vi "Omniax_mDrive_Yonly_2017APXNoBK.vi"() -> ()   [LabVIEW 2015]
uses:
  <vilib>/Utility/file.llb/Read From Spreadsheet File (I64).vi
  <vilib>/Instr/_visa.llb/VISA Configure Serial Port (Instr).vi
  <userlib>/caLab/Private/Get_PV.vi
  Omniax_mDrive_GNDGlobal.vi
  <userlib>/caLab/Private/Put_DBL_PV.vi
  <vilib>/Utility/file.llb/Write To Spreadsheet File (I64).vi
  <vilib>/Utility/file.llb/Write To Spreadsheet File (string).vi
  <vilib>/Utility/file.llb/Read From Spreadsheet File (string).vi
panel:
  out "Z<350?":bool
  out "read buffer":string
  out "sample NC":bool
  in  "APX:MXYZR_STOP":bool
  in  "APX:MY_VLC_RQ":dbl min=0.0 max=0.1 step=0.01
  in  "APX:MY_RQ":dbl min=-3.0 max=2.0
  in  "Y Velocity SP step/sec":i32 min=1 max=12800
  in  "Y Step SP":i32=-20000 min=-2304000 max=2304000 step=500
  out "Y Step PV":i32 max=2000
  out "Boolean":bool
  out "PR P":string
  in  "V5 position 15360000":i32
  out "R Velocity MVdeg/sec":dbl format="%.3f"
  out "R Position MV deg":dbl
  out "Z Velocity MV mm/sec":dbl format="%.3f"
  out "Z Position MV mm":dbl
  out "Y Velocity MV mm/sec":dbl format="%.3f"
  out "Y Position MV mm":dbl
  out "X Velocity MV mm/sec":dbl format="%.3f"
  out "X Position MV mm":dbl
  out "Presets":i32[][](array[numeric])
  in  "stop":bool
  in  "Tab Control 3":enum32{"Status", "Reset"}(tab)
  out "APX:Y_LIM":bool
  out "APX:MY_MVG":bool
  out "APX:MY_RDY":bool
  in  "Reset Y Position mm":dbl
  out "Reset Y Motor Steps":i32
  in  "Reset":bool
  in  "Clear ZY":bool
  out "R Backlash steps/sec":i32
  out "R Backlash":i32
  out "R Holding Current %":i32
  out "R Run Current %":i32
  out "R velocity PV step/sec":i32
  out "Z Backlash steps/sec":i32
  out "Z Backlash":i32
  out "Z Holding Current %":i32
  out "Z Run Current %":i32
  out "Z  velocity PV step/sec":i32
  out "X velocity PV step/sec":i32
  out "X Backlash steps/sec":i32
  out "X Backlash":i32
  out "X Holding Current %":i32
  out "X Run Current %":i32
  out "Y Backlash steps/sec":i32
  out "Y Backlash":i32
  out "Y Holding Current %":i32
  out "Y Run Current %":i32
  out "APX:MY_PV":dbl
  out "Y offset mm":dbl
  out "Y mm/rev":dbl
  out "Y steps/rev":u32
  out "Y velocity PV step/sec":i32
  out "Y MINPOS":i32=-94296
  out "Y MAXPOS":i32=-34296
  out "Y COM PORT":refnum<visa-resource-name>="COM5"
  # "APX:MY"
  # "Goto position"
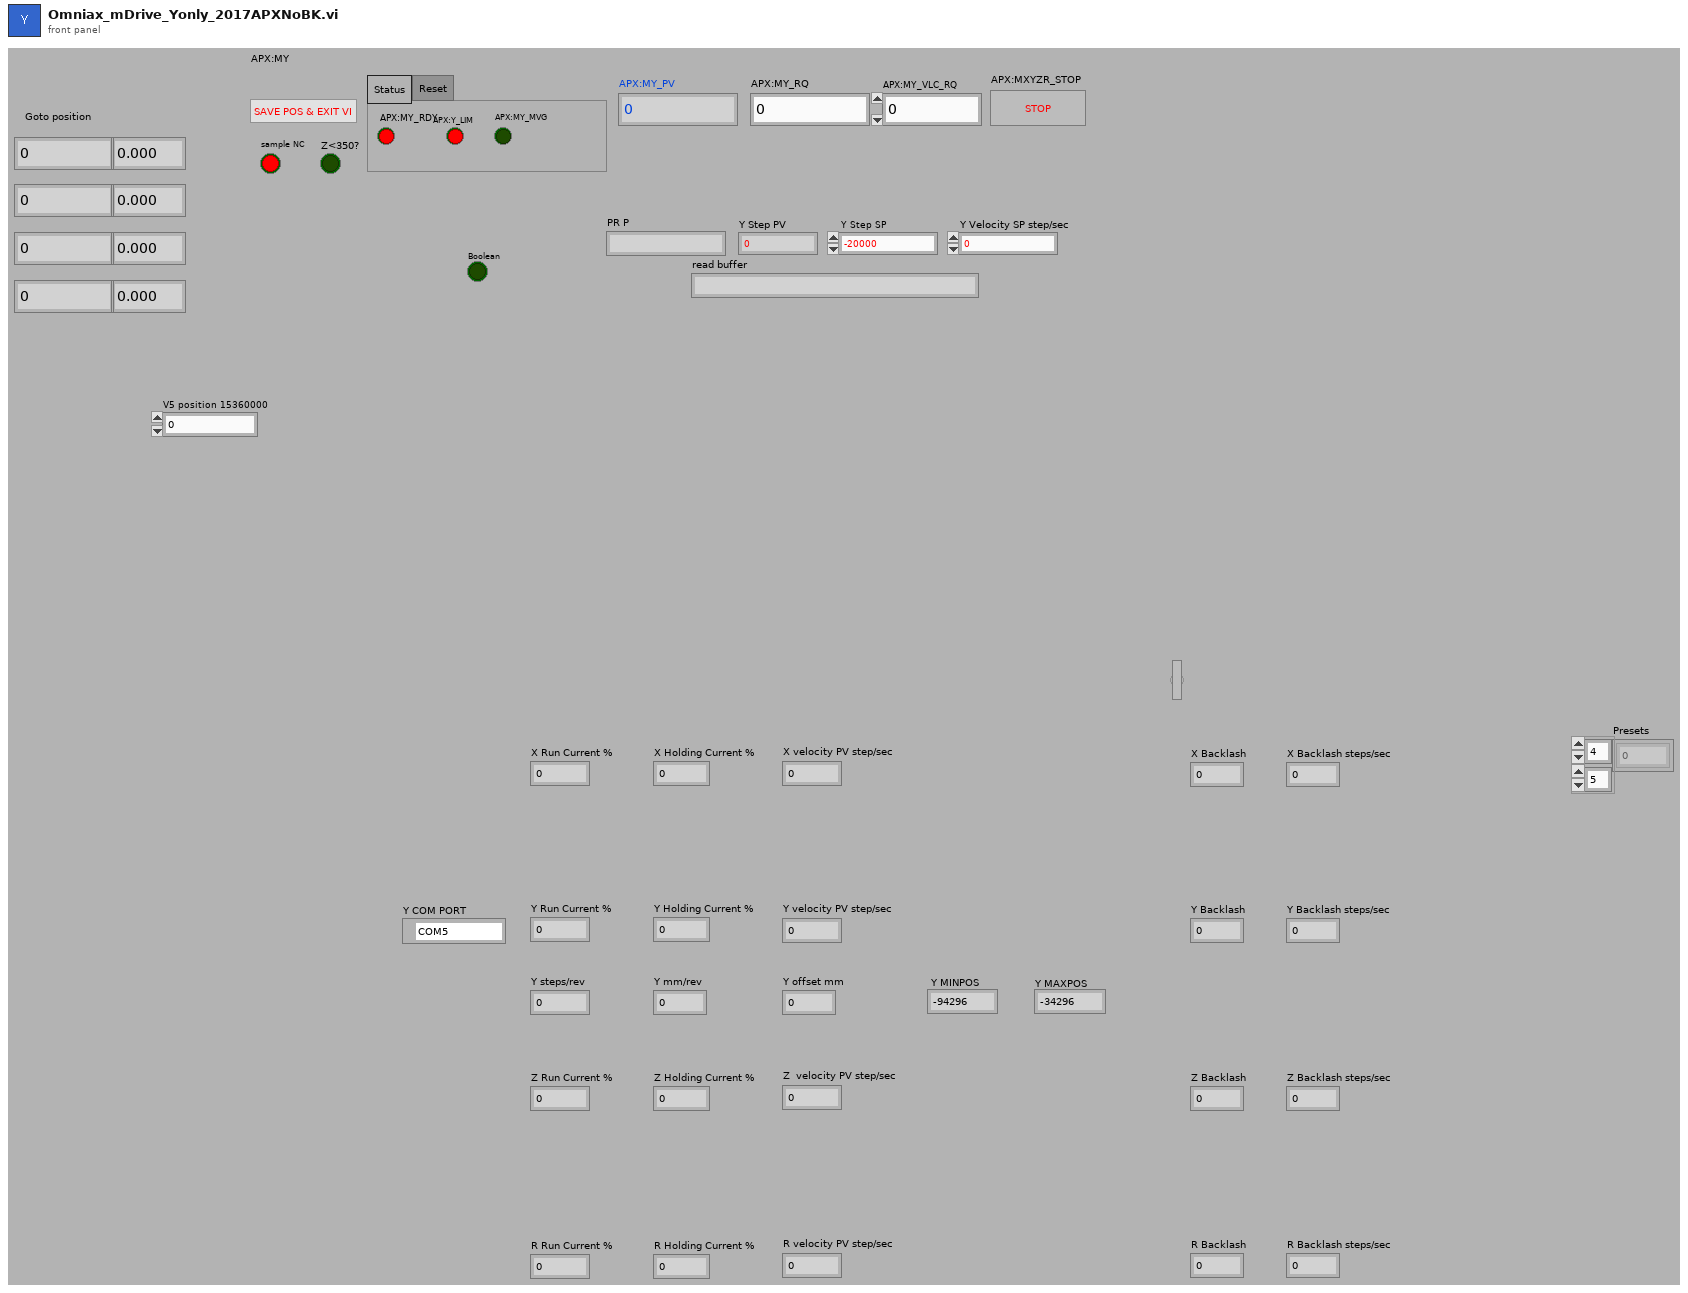
[diagram p1: front panel]
types:
  T1 = enum16{"Stop", "Reset", "Run Current", "Holding Current", "Accel Rate", "Decel Rate", "Move to Relative Position", "Move to Absolute Position", "Echo Mode", "Print Parameter", "Send String", "Microstep Resolution", "Set Current Position", "Max Velocity"}
  T2 = cluster{"first row[0]":i64, "first row[1]":i64, "first row[2]":i64, "first row[3]":i64, "first row[4]":i64, "first row[5]":i64, "first row[6]":i64, "first row[7]":i64, "first row[8]":i64}
  T3 = enum8{"Enabled", "Disabled", "Disabled and Grayed Out"}
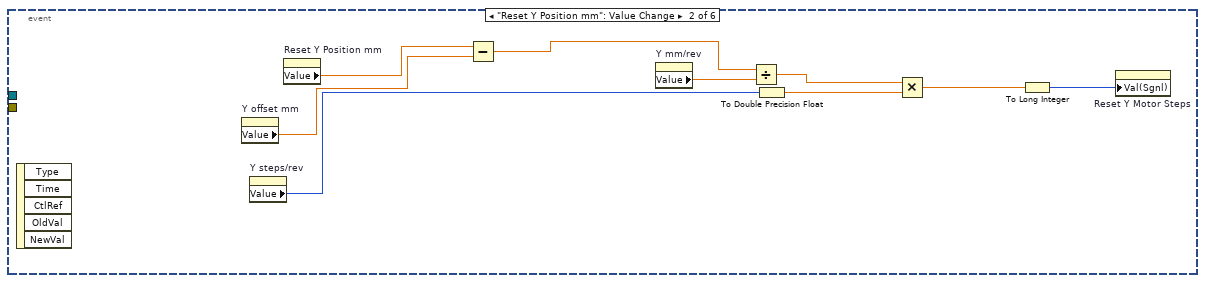
[diagram p13: hidden frame]
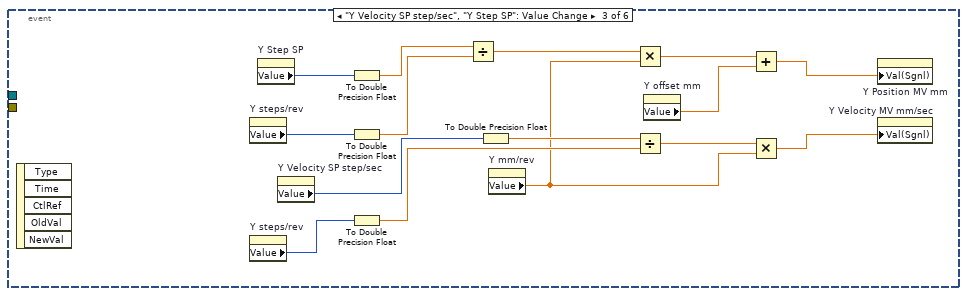
[diagram p14: hidden frame]
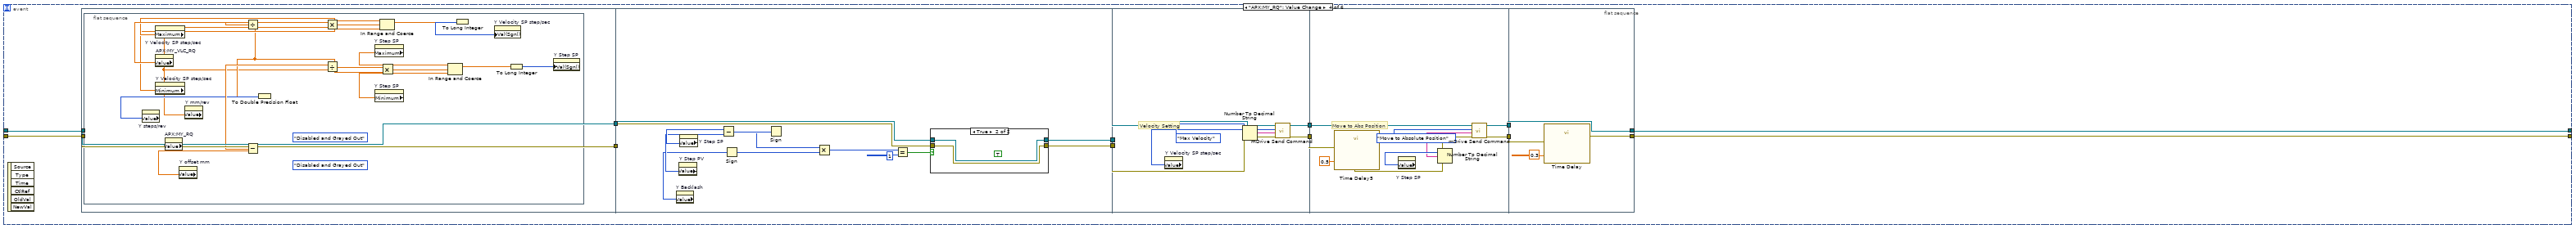
[diagram p15: hidden frame]
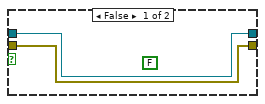
[diagram p16: hidden frame]
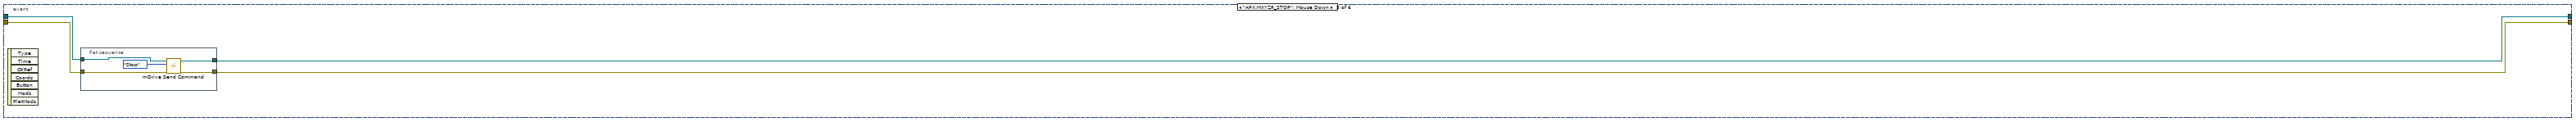
[diagram p17: hidden frame]
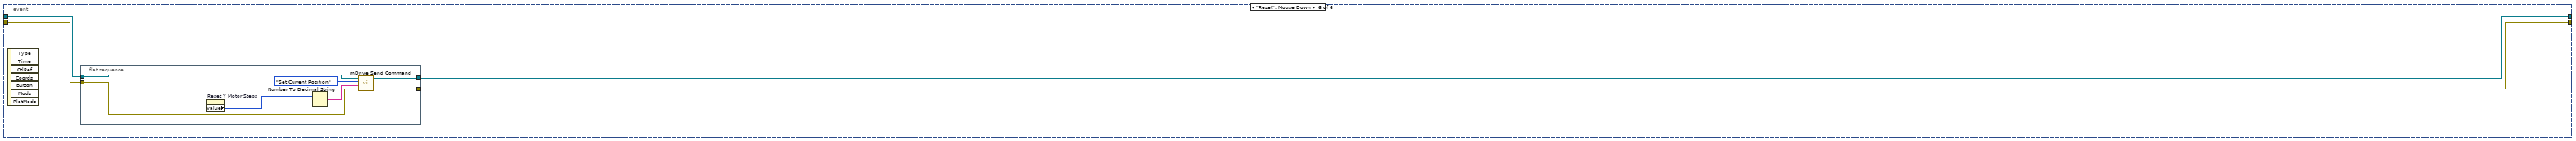
[diagram p18: hidden frame]
diagram:
  (unwired) 6144000 ("upper limit")
  (unwired) -6144000 ("lower limit")
  (unwired) 102400000 ("upper limit")
  (unwired) 0 ("lower limit")
  n1 = flat-sequence {
    tunnel: [w27] -> w10
    tunnel: [w26] -> w9
    tunnel: [w39] -> w14
    tunnel: [w37] -> w12
    tunnel: w10 -> [w36]
    tunnel: w9 -> [w38]
    tunnel: w14 -> [w46]
    tunnel: [w51] -> w13
    tunnel: w12 -> [w44]
    tunnel: [w50] -> w11
    tunnel: [w60] -> w21
    tunnel: [w62] -> w19
    tunnel: w13 -> [w61]
    tunnel: w11 -> [w63]
    tunnel: w21 -> [w70]
    tunnel: [w69] -> w20
    tunnel: w19 -> [w67]
    tunnel: [w68] -> w18
    tunnel: [w80] -> w23
    tunnel: [w81] -> w22
    tunnel: w20 -> [w79]
    tunnel: w18 -> [w78]
    tunnel: w23 -> [w91]
    tunnel: w22 -> [w90]
    tunnel: [w93] -> w17
    tunnel: [w92] -> w16
    tunnel: [w87] -> w15
    tunnel: [w98] -> w24
    tunnel: [w99] -> w25
    tunnel: w17 -> [w99]
    tunnel: w16 -> [w98]
    tunnel: w15 -> [w94]
    frame #0 {
      w34 = refnum<visa-resource-name> "COM13" ("COM PORT")
      w32 = u16 0 items=["None", "XON/XOFF", "RTS/CTS", "XON/XOFF & RTS/CTS", "DTR/DSR", "XON/XOFF & DTR/DSR"] ("flow control (0:none)")
      w31 = u16 10 items=["1.0"=10, "1.5"=15, "2.0"=20] ("stop bits (10: 1 bit)")
      # "Stop bits"
      n2 = call-poly "VISA Configure Serial Port"("VISA resource name"=w34, "timeout (10sec)"=u32 10000, "baud rate (9600)"=u32 9600, "data bits (8)"=u16 8, "parity (0:none)"=enum16{"None", "Odd", "Even", "Mark", "Space"}."None", "stop bits (10: 1 bit)"=w31, "flow control (0:none)"=w32) -> ("VISA resource name out"=w27:refnum<visa-resource-name>, "error out"=w26:errorcluster)  [unwired: 7 in]
      "Y COM PORT" <- w34
    }
    frame #1 {
      n3 = VISA Flush I/O Buffer(VISA resource name=w36) -> (VISA resource name out=w35:refnum<visa-resource-name>)  [unwired: 2 in, 1 out]
      n4 = call "mDrive Send Command.vi"("error in (no error)"=w38, "Extra"="EM 2", "Command"=T1."Send String", "VISA resource name"=w35) -> ("error out"=w37:errorcluster, "VISA resource name out"=w39:refnum<visa-resource-name>)  [unwired: 3 in, 1 out]
    }
    frame #2 {
      n5 = Number To Decimal String(number=1000000) -> (decimal integer string=w52:string)  [unwired: 1 in]
      n6 = call "mDrive Send Command.vi"("error in (no error)"=w44, "Extra"="EE 0", "Command"=T1."Send String", "VISA resource name"=w46) -> ("error out"=w43:errorcluster, "read buffer"=→"read buffer":string, "VISA resource name out"=w45:refnum<visa-resource-name>)  [unwired: 3 in]
      n7 = call "mDrive Send Command.vi"("error in (no error)"=w43, "Extra"=w52, "Command"=T1."Accel Rate", "VISA resource name"=w45) -> ("error out"=w49:errorcluster, "VISA resource name out"=w56:refnum<visa-resource-name>)  [unwired: 3 in, 1 out]
      n8 = call "mDrive Send Command.vi"("error in (no error)"=w49, "Extra"=w52, "Command"=T1."Decel Rate", "VISA resource name"=w56) -> ("error out"=w50:errorcluster, "VISA resource name out"=w51:refnum<visa-resource-name>)  [unwired: 3 in, 1 out]
    }
    frame #3 {
      # "Run Current %"
      n9 = property on="Y Run Current %" class="DigNum (strict)"() -> ("Value"=w58:i32)  [unwired: 2 in, 2 out]
      n10 = Number To Decimal String(number=w58) -> (decimal integer string=w59:string)  [unwired: 1 in]
      n11 = call "mDrive Send Command.vi"("error in (no error)"=w63, "Extra"=w59, "Command"=T1."Run Current", "VISA resource name"=w61) -> ("error out"=w62:errorcluster, "VISA resource name out"=w60:refnum<visa-resource-name>)  [unwired: 3 in, 1 out]
    }
    frame #4 {
      # "Holding Current %"
      n12 = property on="Y Holding Current %" class="DigNum (strict)"() -> ("Value"=w65:i32)  [unwired: 2 in, 2 out]
      n13 = Number To Decimal String(number=w65) -> (decimal integer string=w66:string)  [unwired: 1 in]
      n14 = call "mDrive Send Command.vi"("error in (no error)"=w67, "Extra"=w66, "Command"=T1."Holding Current", "VISA resource name"=w70) -> ("error out"=w68:errorcluster, "VISA resource name out"=w69:refnum<visa-resource-name>)  [unwired: 3 in, 1 out]
    }
    frame #5 {
      # "Velocity Max"
      n15 = property on="Y Velocity SP step/sec" class="DigNum (strict)"() -> ("Value"=w77:i32)  [unwired: 2 in, 2 out]
      n16 = Number To Decimal String(number=w77) -> (decimal integer string=w76:string)  [unwired: 1 in]
      n17 = call "mDrive Send Command.vi"("error in (no error)"=w78, "Extra"=w76, "Command"=T1."Max Velocity", "VISA resource name"=w79) -> ("error out"=w74:errorcluster, "VISA resource name out"=w84:refnum<visa-resource-name>)  [unwired: 3 in, 1 out]
      n18 = call "mDrive Send Command.vi"("error in (no error)"=w74, "Extra"="VM", "Command"=T1."Print Parameter", "VISA resource name"=w84) -> ("error out"=w81:errorcluster, "read buffer"=w82:string, "VISA resource name out"=w80:refnum<visa-resource-name>)  [unwired: 3 in]
      n19 = Decimal String To Number(string=w82, offset=0) -> (number=w75:i32)  [unwired: 1 in, 1 out]
      n20 = property on="Y scan velocity MV step/sec" class="DigNum (strict)"("Val(Sgnl)"=w75) -> ()  [unwired: 2 in, 2 out]
    }
    frame #6 {
      # "PRINT POSITION"
      n21 = call "mDrive Send Command.vi"("error in (no error)"=w90, "Extra"="P", "Command"=T1."Print Parameter", "VISA resource name"=w91) -> ("error out"=w92:errorcluster, "read buffer"=w89:string, "VISA resource name out"=w93:refnum<visa-resource-name>)  [unwired: 3 in]
      n22 = Decimal String To Number(string=w89, offset=0) -> (number=w87:i32)  [unwired: 1 in, 1 out]
    }
    frame #7 {
      w96 = -2304000 ("lower limit")
      w97 = 2304000 ("upper limit")
      n23 = property on="Y Step SP" class="DigNum (strict)"("Val(Sgnl)"=w94) -> ()  [unwired: 2 in, 2 out]
      n24 = property on="Y Step SP" class="DigNum (strict)"("Maximum"=w97) -> ()  [unwired: 2 in, 2 out]
      n25 = In Range and Coerce(upper limit=w97, x=w94, lower limit=w96) -> (In Range?=w95:bool)  [unwired: 1 out]
      n26 = property on="Y Step SP" class="DigNum (strict)"("Minimum"=w96) -> ()  [unwired: 2 in, 2 out]
      n27 = property on="APX:Y_LIM" class="Bool (strict)"("Val(Sgnl)"=w95) -> ()  [unwired: 2 in, 2 out]
      "Y MINPOS" <- w96
      "Y MAXPOS" <- w97
    }
  }
  n28 = disable-structure shown="Disabled" {
    frame Disabled {
      w100 = 0 ("dimension size")
      n29 = call-poly <vilib>:"Read From Spreadsheet File.vi"("file path (dialog if empty)"=path "S:/SSE/IMS/PRESET.TXT") -> ("all rows"=w106:string[][])  [unwired: 6 in, 4 out]
      n30 = Transpose 2D Array(2D array=w106) -> (transposed array=w107:string[][])
      n31 = Delete From Array(array=w107, index (row)=0) -> (deleted portion=w108:string[], array with subset deleted=w110:string[][])  [unwired: 2 in]
      n32 = Transpose 2D Array(2D array=w110) -> (transposed array=w111:string[][])
      n33 = Decimal String To Number(string=w111) -> (number=w109:i32[][])  [unwired: 2 in, 1 out]
      n34 = Initialize Array(w100, w100, 4 ("dimension size")) -> (w103:i32[][])
      n35 = Build Array (concatenate)(w103, w109) -> (→"Presets":i32[][])
    }
    frame Enabled {
    }
  }
  n36 = disable-structure shown="Disabled" {
    disable-tunnel: [w113 _] -> _
    disable-tunnel: [w112 _] -> _
    frame Disabled {
      n37 = call "DigitalIO_sub_V5_MON.vi"() -> ("CL"=w112:bool, "OP"=w113:bool)  [unwired: 8 in]
    }
    frame Enabled {
    }
  }
  n38 = disable-structure shown="Disabled" {
    frame Disabled {
      n39 = flat-sequence {
        frame #0 {
          w114 = FALSE ("Value (Signaling)")
          w117 = FALSE ("Value (Signaling)")
          w120 = FALSE ("Value (Signaling)")
          w121 = FALSE ("Value (Signaling)")
          "Z Backlash steps/sec" <- 25600 ("Z Backlash steps/sec")
          "Z Backlash" <- -51200 ("Z Backlash")
          "X Backlash steps/sec" <- 25600 ("Value (Signaling)")
          "X Backlash" <- 10240 ("Backlash2")
          "Y Backlash" <- -10240 ("Backlash2")
          "Y Backlash steps/sec" <- 25600 ("Value (Signaling)")
          "R Backlash steps/sec" <- 6400 ("R Backlash steps/sec")
          "R Backlash" <- -12800 ("R Backlash")
        }
      }
    }
    frame Enabled {
    }
  }
  n40 = flat-sequence {
    frame #0 {
      "Z Holding Current %" <- 20 ("Z Holding Current %")
      "Z Run Current %" <- 40 ("Z Run Current %")
      "X Run Current %" <- 40 ("Run Current %")
      "X Holding Current %" <- 20 ("Holding Current %")
      "Y Run Current %" <- 40 ("Run Current %")
      "Y Holding Current %" <- 20 ("Holding Current %")
      "R Holding Current %" <- 15 ("R Holding Current %")
      "R Run Current %" <- 80 ("R Run Current %")
    }
  }
  n41 = flat-sequence {
    frame #0 {
      w136 = 0.2 ("MM/rev")
      w139 = u32 51200 ("step/rev")
      w134 = 12800 ("Value (Signaling)")
      n42 = To Double Precision Float(number=w134) -> (double precision float=w140:dbl)
      n43 = To Double Precision Float(number=w139) -> (double precision float=w138:dbl)
      n44 = property on="Y Velocity SP step/sec" class="DigNum (strict)"("Val(Sgnl)"=w134) -> ()  [unwired: 2 in, 2 out]
      n45 = property on="Y Velocity SP step/sec" class="DigNum (strict)"("Minimum"=1.0 ("Data Entry Limits:Minimum")) -> ()  [unwired: 2 in, 2 out]
      n46 = Divide(x=w140, y=w138) -> (x/y=w135:dbl)
      n47 = property on="Y Velocity SP step/sec" class="DigNum (strict)"("Maximum"=w140) -> ()  [unwired: 2 in, 2 out]
      n48 = Multiply(x=w135, y=w136) -> (x*y=w137:dbl)
      n49 = property on="APX:MY_VLC_RQ" class="DigNum (strict)"("Val(Sgnl)"=w137) -> ()  [unwired: 2 in, 2 out]
      "Y offset mm" <- 0.0 ("offset")
      "Y steps/rev" <- w139
      "Y mm/rev" <- w136
    }
  }
  n50 = property on="V5 position 15360000" class="DigNum (strict)"("Value"=15360000 ("V5 position 15360000")) -> ()  [unwired: 2 in, 2 out]
  n51 = call-poly <vilib>:"Read From Spreadsheet File.vi"("file path (dialog if empty)"=path "S:/SSE/IMS/POSY.TXT") -> ("first row"=w5:i64[])  [unwired: 6 in, 4 out]
  n52 = Array To Cluster(array=w5) -> (cluster=w4:T2)
  n53 = Unbundle(w4) -> ("first row[0]"=w1:i64)  [unwired: 8 out]
  n54 = property on="Reset Y Motor Steps" class="DigNum (strict)"("Val(Sgnl)"=w1) -> ()  [unwired: 2 in, 2 out]
  n55 = while {
    tunnel: w25 -> [w144]
    tunnel: w24 -> [w147]
    tunnel: [w148] -> w7
    tunnel: [w146] -> w8
    stop <- "stop" stop-if-true
    n56 = disable-structure shown="Disabled" {
      frame Disabled {
        n57 = flat-sequence {
          frame #0 {
            n58 = call "DAQ Assistant"("number of samples"=100) -> ("data"=w154:dynamicdata)  [unwired: 16 in, 2 out]
            n59 = call "Convert from Dynamic Data"("Dynamic Data Type"=w154) -> ("Array"=w153:dbl[])  [unwired: 3 in]
            n60 = Add Array Elements(numeric array=w153) -> (sum=w152:dbl)
            n61 = Absolute Value(x=w152) -> (abs(x)=w149:dbl)
            n62 = Less?(x=w149, y=1.0) -> (x < y?=w150:bool)
          }
        }
      }
      frame Enabled {
      }
    }
    n63 = event shown="[0] Timeout" {
      selector: _ -> [_ _ _ _ _ _]
      dyn-events: _ -> [_ _ _ _ _ _]
      timeout: 100 -> [_ _ _ _ _ _]
      tunnel: w147 -> [w167 _ _ w365 w433 w442]
      tunnel: [w182 _ _ w371 w431 w440] -> w148
      tunnel: w144 -> [w169 _ _ w366 w434 w443]
      tunnel: [w181 _ _ w372 w432 w441] -> w146
      event Timeout {
        n64 = event-data() -> ()  [unwired: 1 in, 2 out]
        n65 = flat-sequence {
          tunnel: w166 -> [w230]
          tunnel: w168 -> [w229]
          tunnel: [w235] -> w180
          tunnel: [w211] -> w178
          tunnel: [w222] -> w176
          tunnel: [w202] -> w174
          tunnel: [w198] -> w165
          tunnel: w180 -> [w247]
          tunnel: [w247] -> w179
          tunnel: w178 -> [w246]
          tunnel: [w246] -> w177
          tunnel: w176 -> [w245]
          tunnel: [w245] -> w175
          tunnel: w174 -> [w244]
          tunnel: [w244] -> w170
          tunnel: w165 -> [w243]
          tunnel: [w243] -> w164
          tunnel: w179 -> [w251]
          tunnel: [w252] -> w173
          tunnel: w177 -> [w254]
          tunnel: [w253] -> w172
          tunnel: w175 -> [w250]
          tunnel: [w249] -> w171
          tunnel: w170 -> [w249]
          tunnel: w164 -> [w248]
          tunnel: [w248] -> w163
          tunnel: w173 -> [w266]
          tunnel: w172 -> [w267]
          tunnel: w171 -> [w268]
          tunnel: [w265] -> w182
          tunnel: [w264] -> w181
          tunnel: w163 -> [w262]
          frame #0 {
            w206 = 0.1 ("Delay Time (s)")
            n66 = call "mDrive Send Command.vi"("error in (no error)"=w230, "Extra"="P", "Command"=T1."Print Parameter", "VISA resource name"=w229) -> ("error out"=w228:errorcluster, "read buffer"=w234:string, "VISA resource name out"=w232:refnum<visa-resource-name>)  [unwired: 3 in]
            "PR P" <- w234
            n67 = Decimal String To Number(string=w234, offset=0) -> (number=w213:i32)  [unwired: 1 in, 1 out]
            n68 = call "Time Delay4"("error in (no error)"=w228, "Delay Time (s)"=w206) -> ("error out"=w227:errorcluster)  [unwired: 9 in]
            n69 = property on="Y Step SP" class="DigNum (strict)"() -> ("Maximum"=w224:dbl)  [unwired: 2 in, 2 out]
            n70 = property on="Y Step SP" class="DigNum (strict)"() -> ("Minimum"=w226:dbl)  [unwired: 2 in, 2 out]
            n71 = To Long Integer(number=w213) -> (32bit integer=w214:i32)
            n72 = property on="Y Step PV" class="DigNum (strict)"("Val(Sgnl)"=w214) -> ()  [unwired: 2 in, 2 out]
            n73 = To Long Integer(number=w224) -> (32bit integer=w223:i32)
            n74 = To Long Integer(number=w226) -> (32bit integer=w225:i32)
            n75 = property on="Y steps/rev" class="DigNum (strict)"() -> ("Value"=w220:u32)  [unwired: 2 in, 2 out]
            n76 = In Range and Coerce(upper limit=w223, x=w214, lower limit=w225) -> (In Range?=w222:bool)  [unwired: 1 out]
            n77 = To Double Precision Float(number=w214) -> (double precision float=w215:dbl)
            n78 = To Double Precision Float(number=w220) -> (double precision float=w221:dbl)
            n79 = disable-structure shown="Disabled" {
              disable-tunnel: [w242 _] -> w235
              disable-tunnel: w232 -> [w241 _]
              disable-tunnel: [w240 _] -> w231
              disable-tunnel: w227 -> [w239 _]
              disable-tunnel: T1."Print Parameter" ("Command") -> [w238 _]
              disable-tunnel: "MV" ("Extra") -> [w237 _]
              disable-tunnel: [w236 _] -> w199
              frame Disabled {
                n80 = call "mDrive Send Command.vi"("error in (no error)"=w239, "Extra"=w237, "Command"=w238, "VISA resource name"=w241) -> ("error out"=w240:errorcluster, "read buffer"=w236:string, "VISA resource name out"=w242:refnum<visa-resource-name>)  [unwired: 3 in]
              }
              frame Enabled {
              }
            }
            n81 = property on="APX:Y_LIM" class="Bool (strict)"("Val(Sgnl)"=w222) -> ()  [unwired: 2 in, 2 out]
            n82 = Divide(x=w215, y=w221) -> (x/y=w219:dbl)
            n83 = property on="Y mm/rev" class="DigNum (strict)"() -> ("Value"=w218:dbl)  [unwired: 2 in, 2 out]
            n84 = call "Time Delay3"("error in (no error)"=w231, "Delay Time (s)"=w206) -> ("error out"=w211:errorcluster)  [unwired: 9 in]
            n85 = Multiply(x=w219, y=w218) -> (x*y=w217:dbl)
            n86 = Decimal String To Number(string=w199, offset=0 ("offset (0)")) -> (number=w205:i32)  [unwired: 1 in, 1 out]
            n87 = Not Equal?(x=w199, y="") -> (x != y?=w200:bool)
            n88 = property on="APX:MY_RDY" class="Bool (strict)"("Val(Sgnl)"=w200) -> ()  [unwired: 2 in, 2 out]
            n89 = property on="Y offset mm" class="DigNum (strict)"() -> ("Value"=w216:dbl)  [unwired: 2 in, 2 out]
            n90 = Number To Boolean Array(number=w205) -> (Boolean array=w204:bool[])
            n91 = Add(x=w217, y=w216) -> (x+y=w198:dbl)
            n92 = Index Array(array=w204, index=0) -> (element=w202:bool)
            n93 = property on="APX:MY_PV" class="DigNum (strict)"("Val(Sgnl)"=w198) -> ()  [unwired: 2 in, 2 out]
            n94 = property on="APX:MY_MVG" class="Bool (strict)"("Val(Sgnl)"=w202) -> ()  [unwired: 2 in, 2 out]
          }
          frame #1 {
          }
          frame #2 {
            n95 = case shown="False" w250 {
              tunnel: w251 -> [w257 w261]
              tunnel: [w258 w261] -> w252
              tunnel: [w259 w260] -> w253
              tunnel: w254 -> [w256 w260]
              frame False {
                n96 = call "mDrive Send Command.vi"("error in (no error)"=w256, "Command"=T1."Stop", "VISA resource name"=w257) -> ("error out"=w259:errorcluster, "VISA resource name out"=w258:refnum<visa-resource-name>)  [unwired: 4 in, 1 out]
              }
              frame True {
              }
            }
            "Boolean" <- w250
          }
          frame #3 {
            n97 = disable-structure shown="Disabled" {
              disable-tunnel: w268 -> [w274 _]
              disable-tunnel: w267 -> [w272 _]
              disable-tunnel: w266 -> [w271 _]
              disable-tunnel: [w270 _] -> w265
              disable-tunnel: [w269 _] -> w264
              frame Disabled {
                n98 = Implies(1:w274) -> (0:w273:bool, 2:w275:bool)
                n99 = case shown="False" w273 {
                  tunnel: w272 -> [w282 w335]
                  tunnel: w271 -> [w281 w336]
                  tunnel: [w280 w335] -> w270
                  tunnel: [w279 w336] -> w269
                  frame False {
                    # "Backlash"
                    n100 = flat-sequence {
                      tunnel: [w297] -> w294
                      tunnel: [w299] -> w293
                      tunnel: [w298] -> w292
                      tunnel: w282 -> [w296]
                      tunnel: w281 -> [w295]
                      tunnel: w294 -> [w307]
                      tunnel: [w307] -> w291
                      tunnel: w293 -> [w306]
                      tunnel: w292 -> [w305]
                      tunnel: [w304] -> w290
                      tunnel: [w303] -> w289
                      tunnel: [w302] -> w278
                      tunnel: w291 -> [w317]
                      tunnel: w290 -> [w316]
                      tunnel: w289 -> [w314]
                      tunnel: [w315] -> w288
                      tunnel: [w314] -> w287
                      tunnel: [w313] -> w284
                      tunnel: [w312] -> w283
                      tunnel: w278 -> [w312]
                      tunnel: w288 -> [w328]
                      tunnel: w287 -> [w321]
                      tunnel: [w328] -> w286
                      tunnel: [w327] -> w285
                      tunnel: w284 -> [w327]
                      tunnel: w283 -> [w323]
                      tunnel: [w322] -> w276
                      tunnel: w286 -> [w332]
                      tunnel: w285 -> [w331]
                      tunnel: [w330] -> w280
                      tunnel: [w329] -> w277
                      tunnel: w276 -> [w329]
                      tunnel: [w334] -> w279
                      tunnel: w277 -> [w334]
                      frame #0 {
                        n101 = property on="Y Backlash steps/sec" class="DigNum (strict)"() -> ("Value"=w297:i32)  [unwired: 2 in, 2 out]
                        n102 = Number To Decimal String(number=w297) -> (decimal integer string=w300:string)  [unwired: 1 in]
                        n103 = call "mDrive Send Command.vi"("error in (no error)"=w296, "Extra"=w300, "Command"=T1."Max Velocity", "VISA resource name"=w295) -> ("error out"=w298:errorcluster, "VISA resource name out"=w299:refnum<visa-resource-name>)  [unwired: 3 in, 1 out]
                      }
                      frame #1 {
                        n104 = property on="Y Backlash" class="DigNum (strict)"() -> ("Value"=w302:i32)  [unwired: 2 in, 2 out]
                        n105 = Number To Decimal String(number=w302) -> (decimal integer string=w308:string)  [unwired: 1 in]
                        n106 = call "mDrive Send Command.vi"("error in (no error)"=w305, "Extra"=w308, "Command"=T1."Move to Relative Position", "VISA resource name"=w306) -> ("error out"=w304:errorcluster, "VISA resource name out"=w303:refnum<visa-resource-name>)  [unwired: 3 in, 1 out]
                      }
                      frame #2 {
                        n107 = To Double Precision Float(number=w312) -> (double precision float=w310:dbl)
                        n108 = To Double Precision Float(number=w317) -> (double precision float=w319:dbl)
                        n109 = Absolute Value(x=w310) -> (abs(x)=w311:dbl)
                        n110 = Divide(x=w311, y=w319) -> (x/y=w320:dbl)
                        n111 = Add(x=w320, y=0.3) -> (x+y=w313:dbl)
                        n112 = call "Time Delay8"("error in (no error)"=w316, "Delay Time (s)"=w313) -> ("error out"=w315:errorcluster)  [unwired: 9 in]
                      }
                      frame #3 {
                        n113 = Negate(x=w323) -> (-x=w324:i32)
                        n114 = Number To Decimal String(number=w324) -> (decimal integer string=w325:string)  [unwired: 1 in]
                        n115 = call "mDrive Send Command.vi"("Extra"=w325, "Command"=T1."Move to Relative Position", "VISA resource name"=w321) -> ("VISA resource name out"=w322:refnum<visa-resource-name>)  [unwired: 4 in, 2 out]
                      }
                      frame #4 {
                        n116 = call "Time Delay2"("error in (no error)"=w332, "Delay Time (s)"=w331) -> ("error out"=w330:errorcluster)  [unwired: 9 in]
                      }
                      frame #5 {
                        w333 = FALSE ("Value (Signaling)")
                      }
                    }
                  }
                  frame True {
                  }
                }
              }
              frame Enabled {
              }
            }
            n117 = call-poly <userlib>:"CaLabPut.vi"("Value"=w262, "PV Name"="APX:OmniaxY") -> ()  [unwired: 6 in, 4 out]
          }
        }
        n118 = global read "Omniax_mDrive_GNDGlobal.vi" "sample NC"() -> (→"sample NC":bool)
        n119 = disable-structure shown="Disabled" {
          frame Disabled {
            n120 = Divide() -> (x=w190:dbl, y=w191:dbl, x/y=w192:dbl)
            n121 = Inverse Tangent(1:w192) -> (0:w193:dbl)
            n122 = Divide(x=w193, y=6.283185307179586) -> (x/y=w194:dbl)
            n123 = Multiply(x=360.0, y=w194) -> (x*y=w197:dbl)
          }
          frame Enabled {
          }
        }
        n124 = call-poly "CaLabGet.vi"("PV Name"="APX:OmniaxZ") -> ("1rst Value (number)"=w161:dbl)  [unwired: 8 in, 6 out]
        n125 = Less?(x=w161, y=350.0) -> (x < y?=w158:bool)
        "Z<350?" <- w158
        n126 = And(x=w158, y=TRUE) -> (x .and. y?=w159:bool)
        n127 = case shown="False" w159 {
          tunnel: w169 -> [w187 w188]
          tunnel: w167 -> [w185 w189]
          tunnel: [w184 w189] -> w166
          tunnel: [w183 w188] -> w168
          frame False {
            n128 = call "mDrive Send Command.vi"("error in (no error)"=w185, "Command"=T1."Stop", "VISA resource name"=w187) -> ("error out"=w184:errorcluster, "VISA resource name out"=w183:refnum<visa-resource-name>)  [unwired: 4 in, 1 out]
          }
          frame True {
          }
        }
      }
      event "Reset Y Position mm": Value Change {
        n129 = event-data() -> ()  [unwired: 1 in, 5 out]
        n130 = property on="Y offset mm" class="DigNum (strict)"() -> ("Value"=w337:dbl)  [unwired: 2 in, 2 out]
        n131 = property on="Y steps/rev" class="DigNum (strict)"() -> ("Value"=w339:u32)  [unwired: 2 in, 2 out]
        n132 = property on="Reset Y Position mm" class="DigNum (strict)"() -> ("Value"=w345:dbl)  [unwired: 2 in, 2 out]
        n133 = Subtract(x=w345, y=w337) -> (x-y=w344:dbl)
        n134 = property on="Y mm/rev" class="DigNum (strict)"() -> ("Value"=w338:dbl)  [unwired: 2 in, 2 out]
        n135 = Divide(x=w344, y=w338) -> (x/y=w343:dbl)
        n136 = To Double Precision Float(number=w339) -> (double precision float=w342:dbl)
        n137 = Multiply(x=w343, y=w342) -> (x*y=w341:dbl)
        n138 = To Long Integer(number=w341) -> (32bit integer=w340:i32)
        n139 = property on="Reset Y Motor Steps" class="DigNum (strict)"("Val(Sgnl)"=w340) -> ()  [unwired: 2 in, 2 out]
      }
      event "Y Velocity SP step/sec", "Y Step SP": Value Change {
        n140 = event-data() -> ()  [unwired: 1 in, 5 out]
        n141 = property on="Y steps/rev" class="DigNum (strict)"() -> ("Value"=w348:u32)  [unwired: 2 in, 2 out]
        n142 = property on="Y steps/rev" class="DigNum (strict)"() -> ("Value"=w355:u32)  [unwired: 2 in, 2 out]
        n143 = property on="Y Step SP" class="DigNum (strict)"() -> ("Value"=w350:i32)  [unwired: 2 in, 2 out]
        n144 = property on="Y Velocity SP step/sec" class="DigNum (strict)"() -> ("Value"=w357:i32)  [unwired: 2 in, 2 out]
        n145 = To Double Precision Float(number=w350) -> (double precision float=w351:dbl)
        n146 = To Double Precision Float(number=w348) -> (double precision float=w354:dbl)
        n147 = To Double Precision Float(number=w355) -> (double precision float=w360:dbl)
        n148 = Divide(x=w351, y=w354) -> (x/y=w353:dbl)
        n149 = To Double Precision Float(number=w357) -> (double precision float=w358:dbl)
        n150 = property on="Y mm/rev" class="DigNum (strict)"() -> ("Value"=w346:dbl)  [unwired: 2 in, 2 out]
        n151 = Multiply(x=w353, y=w346) -> (x*y=w352:dbl)
        n152 = Divide(x=w358, y=w360) -> (x/y=w359:dbl)
        n153 = property on="Y offset mm" class="DigNum (strict)"() -> ("Value"=w347:dbl)  [unwired: 2 in, 2 out]
        n154 = Add(x=w352, y=w347) -> (x+y=w349:dbl)
        n155 = Multiply(x=w359, y=w346) -> (x*y=w356:dbl)
        n156 = property on="Y Position MV mm" class="DigNum (strict)"("Val(Sgnl)"=w349) -> ()  [unwired: 2 in, 2 out]
        n157 = property on="Y Velocity MV mm/sec" class="DigNum (strict)"("Val(Sgnl)"=w356) -> ()  [unwired: 2 in, 2 out]
      }
      event "APX:MY_RQ": Value Change {
        n158 = event-data() -> ()  [unwired: 1 in, 6 out]
        n159 = flat-sequence {
          tunnel: w365 -> [w373]
          tunnel: w366 -> [w374]
          tunnel: [w374] -> w362
          tunnel: [w373] -> w361
          tunnel: [w396] -> w364
          tunnel: [w395] -> w363
          tunnel: w362 -> [w398]
          tunnel: w361 -> [w397]
          tunnel: [w414] -> w368
          tunnel: [w413] -> w367
          tunnel: w364 -> [w412]
          tunnel: w363 -> [w411]
          tunnel: [w423] -> w370
          tunnel: [w422] -> w369
          tunnel: w368 -> [w421]
          tunnel: w367 -> [w420]
          tunnel: [w429] -> w371
          tunnel: [w430] -> w372
          tunnel: w370 -> [w430]
          tunnel: w369 -> [w428]
          frame #0 {
            (unwired) T3."Disabled and Grayed Out" ("Disabled")
            (unwired) T3."Disabled and Grayed Out" ("Disabled")
            n160 = flat-sequence {
              frame #0 {
                n161 = property on="Y steps/rev" class="DigNum (strict)"() -> ("Value"=w391:u32)  [unwired: 2 in, 2 out]
                n162 = property on="Y Velocity SP step/sec" class="DigNum (strict)"() -> ("Maximum"=w378:dbl)  [unwired: 2 in, 2 out]
                n163 = property on="APX:MY_VLC_RQ" class="DigNum (strict)"() -> ("Value"=w382:dbl)  [unwired: 2 in, 2 out]
                n164 = property on="Y Velocity SP step/sec" class="DigNum (strict)"() -> ("Minimum"=w377:dbl)  [unwired: 2 in, 2 out]
                n165 = property on="APX:MY_RQ" class="DigNum (strict)"() -> ("Value"=w388:dbl)  [unwired: 2 in, 2 out]
                n166 = property on="Y offset mm" class="DigNum (strict)"() -> ("Value"=w389:dbl)  [unwired: 2 in, 2 out]
                n167 = property on="Y mm/rev" class="DigNum (strict)"() -> ("Value"=w375:dbl)  [unwired: 2 in, 2 out]
                n168 = Divide(x=w382, y=w375) -> (x/y=w383:dbl)
                n169 = Subtract(x=w388, y=w389) -> (x-y=w392:dbl)
                n170 = To Double Precision Float(number=w391) -> (double precision float=w376:dbl)
                n171 = Multiply(x=w383, y=w376) -> (x*y=w380:dbl)
                n172 = Divide(x=w392, y=w375) -> (x/y=w393:dbl)
                n173 = property on="Y Step SP" class="DigNum (strict)"() -> ("Maximum"=w385:dbl)  [unwired: 2 in, 2 out]
                n174 = property on="Y Step SP" class="DigNum (strict)"() -> ("Minimum"=w384:dbl)  [unwired: 2 in, 2 out]
                n175 = In Range and Coerce(upper limit=w378, x=w380, lower limit=w377) -> (coerced(x)=w379:dbl)  [unwired: 1 out]
                n176 = Multiply(x=w393, y=w376) -> (x*y=w387:dbl)
                n177 = In Range and Coerce(upper limit=w385, x=w387, lower limit=w384) -> (coerced(x)=w386:dbl)  [unwired: 1 out]
                n178 = To Long Integer(number=w379) -> (32bit integer=w381:i32)
                n179 = property on="Y Velocity SP step/sec" class="DigNum (strict)"("Val(Sgnl)"=w381) -> ()  [unwired: 2 in, 2 out]
                n180 = To Long Integer(number=w386) -> (32bit integer=w390:i32)
                n181 = property on="Y Step SP" class="DigNum (strict)"("Val(Sgnl)"=w390) -> ()  [unwired: 2 in, 2 out]
              }
            }
          }
          frame #1 {
            n182 = property on="Y Backlash" class="DigNum (strict)"() -> ("Value"=w394:i32)  [unwired: 2 in, 2 out]
            n183 = property on="Y Step PV" class="DigNum (strict)"() -> ("Value"=w405:i32)  [unwired: 2 in, 2 out]
            n184 = property on="Y Step SP" class="DigNum (strict)"() -> ("Value"=w406:i32)  [unwired: 2 in, 2 out]
            n185 = Subtract(x=w406, y=w405) -> (x-y=w404:i32)
            n186 = Sign(1:w394) -> (0:w402:i32)
            n187 = Sign(1:w404) -> (0:w403:i32)
            n188 = Multiply(x=w403, y=w402) -> (x*y=w401:i32)
            n189 = Equal?(x=w401, y=1) -> (x = y?=w399:bool)
            n190 = case shown="True" w399 {
              tunnel: w398 -> [w408 w410]
              tunnel: w397 -> [w407 w409]
              tunnel: [w407 w409] -> w396
              tunnel: [w408 w410] -> w395
              frame False {
                (unwired) FALSE ("Value (Signaling)")
              }
              frame True {
                (unwired) TRUE ("Value (Signaling)")
              }
            }
          }
          frame #2 {
            # "Velocity Setting"
            n191 = property on="Y Velocity SP step/sec" class="DigNum (strict)"() -> ("Value"=w415:i32)  [unwired: 2 in, 2 out]
            n192 = Number To Decimal String(number=w415) -> (decimal integer string=w416:string)  [unwired: 1 in]
            n193 = call "mDrive Send Command.vi"("error in (no error)"=w412, "Extra"=w416, "Command"=T1."Max Velocity", "VISA resource name"=w411) -> ("error out"=w413:errorcluster, "VISA resource name out"=w414:refnum<visa-resource-name>)  [unwired: 3 in, 1 out]
          }
          frame #3 {
            # "Move to Abs Position"
            n194 = call "Time Delay5"("error in (no error)"=w420, "Delay Time (s)"=0.5) -> ("error out"=w419:errorcluster)  [unwired: 9 in]
            n195 = property on="Y Step SP" class="DigNum (strict)"() -> ("Value"=w426:i32)  [unwired: 2 in, 2 out]
            n196 = Number To Decimal String(number=w426) -> (decimal integer string=w425:string)  [unwired: 1 in]
            n197 = call "mDrive Send Command.vi"("error in (no error)"=w419, "Extra"=w425, "Command"=T1."Move to Absolute Position", "VISA resource name"=w421) -> ("error out"=w422:errorcluster, "VISA resource name out"=w423:refnum<visa-resource-name>)  [unwired: 3 in, 1 out]
          }
          frame #4 {
            n198 = call "Time Delay"("error in (no error)"=w428, "Delay Time (s)"=0.3) -> ("error out"=w429:errorcluster)  [unwired: 9 in]
          }
        }
      }
      event "APX:MXYZR_STOP": Mouse Down {
        n199 = event-data() -> ()  [unwired: 1 in, 7 out]
        n200 = flat-sequence {
          tunnel: w434 -> [w439]
          tunnel: w433 -> [w438]
          tunnel: [w437] -> w432
          tunnel: [w436] -> w431
          frame #0 {
            n201 = call "mDrive Send Command.vi"("error in (no error)"=w438, "Command"=T1."Stop", "VISA resource name"=w439) -> ("error out"=w436:errorcluster, "VISA resource name out"=w437:refnum<visa-resource-name>)  [unwired: 4 in, 1 out]
          }
        }
      }
      event "Reset": Mouse Down {
        n202 = event-data() -> ()  [unwired: 1 in, 7 out]
        n203 = flat-sequence {
          tunnel: w443 -> [w447]
          tunnel: w442 -> [w446]
          tunnel: [w445] -> w441
          tunnel: [w444] -> w440
          frame #0 {
            n204 = property on="Reset Y Motor Steps" class="DigNum (strict)"() -> ("Value"=w448:i32)  [unwired: 2 in, 2 out]
            n205 = Number To Decimal String(number=w448) -> (decimal integer string=w449:string)  [unwired: 1 in]
            n206 = call "mDrive Send Command.vi"("error in (no error)"=w446, "Extra"=w449, "Command"=T1."Set Current Position", "VISA resource name"=w447) -> ("error out"=w444:errorcluster, "VISA resource name out"=w445:refnum<visa-resource-name>)  [unwired: 3 in, 1 out]
          }
        }
      }
    }
  }
  n207 = flat-sequence {
    tunnel: w8 -> [w457]
    tunnel: w7 -> [w455]
    tunnel: [w453] -> w6
    frame #0 {
      n208 = call "mDrive Send Command.vi"("error in (no error)"=w455, "Extra"="P", "Command"=T1."Print Parameter", "VISA resource name"=w457) -> ("error out"=w452:errorcluster, "read buffer"=w461:string, "VISA resource name out"=w456:refnum<visa-resource-name>)  [unwired: 3 in]
      n209 = Decimal String To Number(string=w461, offset=0) -> (number=w454:i32)  [unwired: 1 in, 1 out]
      n210 = To Long Integer(number=w454) -> (32bit integer=w453:i32)
      n211 = call "Time Delay31"("error in (no error)"=w452) -> ("error out"=w451:errorcluster)  [unwired: 10 in]
      n212 = call "mDrive Send Command.vi"("error in (no error)"=w451, "Command"=T1."Stop", "VISA resource name"=w456) -> ("error out"=w463:errorcluster, "VISA resource name out"=w464:refnum<visa-resource-name>)  [unwired: 4 in, 1 out]
      n213 = VISA Close(VISA resource name=w464, error in (no error)=w463) -> ()  [unwired: 1 out]
    }
  }
  n214 = flat-sequence {
    tunnel: w6 -> [w467]
    frame #0 {
      n215 = Build Array(w467) -> (w465:i32[])
      n216 = call-poly <vilib>:"Write To Spreadsheet File.vi"("1D data"=w465, "file path (dialog if empty)"=path "S:/SSE/IMS/POSY.TXT") -> ()  [unwired: 6 in, 1 out]
    }
    frame #1 {
      n217 = disable-structure shown="Disabled" {
        frame Disabled {
          n218 = property on="Presets" class="Arr (strict)"() -> ("Value"=w474:i32[][])  [unwired: 2 in, 2 out]
          n219 = Number To Decimal String(number=w474) -> (decimal integer string=w468:string[][])  [unwired: 1 in]
          n220 = Transpose 2D Array(2D array=w468) -> (transposed array=w469:string[][])
          n221 = Build Array(w469) -> (w471:string[][][], w470:string[][])
          n222 = Transpose 2D Array(2D array=w471) -> (transposed array=w472:string[][])
          n223 = call-poly <vilib>:"Write To Spreadsheet File.vi"("2D data"=w472, "file path (dialog if empty)"=path "S:/SSE/IMS/PRESET.TXT") -> ()  [unwired: 6 in, 1 out]
        }
        frame Enabled {
        }
      }
    }
  }
